vi "SMTP Email MIME Send Separator.vi"(4 "MIME content-type":string, 5 "translit":string, 6 "binary (F)":bool, 7 "character set":string, 8 "error in (no error)":errorcluster, 9 "name":string, 10 "last (F)":bool, 11 "smtp session":T1) -> (0 "error out":errorcluster, 3 "smtp session out":T1)   [LabVIEW 2011, in "NewNI_SMTPEmail.lvlib"]
uses:
  NewNI_SMTPEmail.lvlib
  SMTP Email Session.ctl
panel:
  in  "buffered tcp connection":refnum<k5>
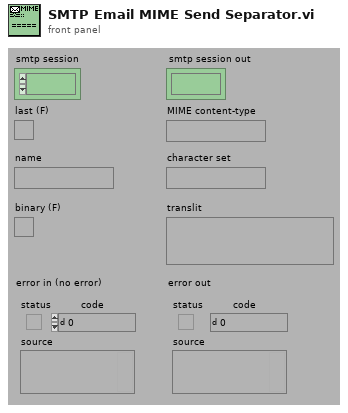
[diagram p1: front panel]
types:
  T1 = typedef "NewNI_SMTPEmail.lvlib/SMTP Email Session.ctl" = refnum<k1>
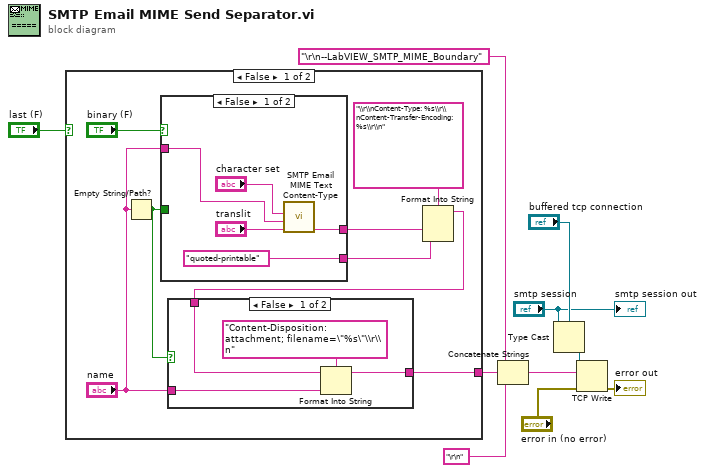
[diagram p0: block diagram]
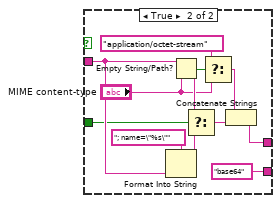
[diagram p3: hidden frame]
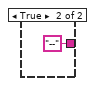
[diagram p4: hidden frame]
diagram:
  n1 = case shown="False" "last (F)" {
    tunnel: [w15 "--"] -> w7
    frame False {
      n2 = Empty String/Path?(string/path="name") -> (empty?=w17:bool)
      n3 = case shown="False" "binary (F)" {
        tunnel: "name" -> [w27 w37]
        tunnel: w17 -> [_ w35]
        tunnel: [w26 w34] -> w13
        tunnel: ["quoted-printable" "base64"] -> w11
        frame False {
          n4 = call "SMTP Email MIME Text Content-Type.vi"("translit"="translit", "name"=w27, "character set"="character set") -> ("MIME content-type"=w26:string)  [unwired: 4 out]
        }
        frame True {
          n5 = Format Into String(format string="; name=\"%s\"", w37) -> (resulting string=w38:string)  [unwired: 2 in, 1 out]
          n6 = Empty String/Path?(string/path="MIME content-type") -> (empty?=w31:bool)
          n7 = Select(t=w37, s=w35, f=w38) -> (s? t:f=w36:string)
          n8 = Select(t="application/octet-stream", s=w31, f="MIME content-type") -> (s? t:f=w32:string)
          n9 = Concatenate Strings(w32, w36) -> (w34:string)
        }
      }
      n10 = Format Into String(format string="\\r\\nContent-Type: %s\\r\\nContent-Transfer-Encoding: %s\\r\\n", w13, w11) -> (resulting string=w12:string)  [unwired: 2 in, 1 out]
      n11 = case shown="False" w17 {
        tunnel: "name" -> [w21 _]
        tunnel: w12 -> [w20 w23]
        tunnel: [w19 w23] -> w15
        frame False {
          n12 = Format Into String(format string="Content-Disposition: attachment; filename=\"%s\"\\r\\n", initial string=w20, w21) -> (resulting string=w19:string)  [unwired: 1 in, 1 out]
        }
        frame True {
        }
      }
    }
    frame True {
    }
  }
  n13 = Concatenate Strings("\r\n--LabVIEW_SMTP_MIME_Boundary", w7, "\r\n") -> (w5:string)
  n14 = Type Cast(type="buffered tcp connection", x="smtp session") -> (*(type *) &x=w2:refnum<k5>)
  n15 = TCP Write(connection ID=w2, data in=w5, error in (no error)="error in (no error)") -> (error out=→"error out":errorcluster)  [unwired: 3 out]
  "smtp session out" <- "smtp session"
